vi "ICR_Hardware_Settings.vi"(8 "error in (no error)":errorcluster, 10 "Use Software Trigger":bool=TRUE, 11 "QMH UI Cluster":variant) -> (0 "error out":errorcluster, 2 "FIFO used":i64, 3 "instrument handle out":refnum<k15>)   [LabVIEW 2015]
doc: "This VI inits a waveform generation session for HSDIO 6541. This is a basic example that shows how to setup the board in order to generate waveforms according to a script. \n\n1. Initialize for a generation session.\n2. Assign specified channels in Channel List for dynamic operation : all = \"\" (default)\n3. Sets the Idle State for when the generation has completed : NO !!\n4. Configure the Sample clock to use the onboard clock, and configure the clock rate.\n5. Set generation mode to Scripted.\n6. Configure the Script Trigger : change to Digital Edge if waiting for an external\n trigger, and link Rising Edge and source trigger commands.\n Use PFI0 with SMB wired to the board, or any PFIxx if connected to accessory."
uses:
  controls/EXPERT_Inputs.ctl
  controls/SOFTWARE_Inputs.ctl
  controls/AO_6711_Inputs.ctl
  controls/AWG_5421_Inputs.ctl
  controls/DIGIT_5122_Inputs.ctl
  <instrlib>/niScope/Controls/niScope trigger source.ctl
  controls/HSDIO_6541_Inputs.ctl
  <instrlib>/niHSDIO/niHSDIO.llb/niHSDIO_ctl Trigger Source Values (Ring).ctl
  controls/SEQUENCE_Inputs.ctl
  controls/TRAPPING_Inputs.ctl
  controls/EXCIT_Inputs.ctl
  controls/DATA_Inputs.ctl
  controls/TIMING_Inputs.ctl
  controls/QMH_UI_Cluster.ctl
  controls/QMH_UI_References.ctl
  controls/QMH_UI_Report.ctl
  controls/QMH_UI_Command.ctl
  controls/QMH_ICR_Command.ctl
  controls/QMH_Status.ctl
  <instrlib>/niHSDIO/niHSDIO.llb/niHSDIO Write Named Waveform (1D U32).vi
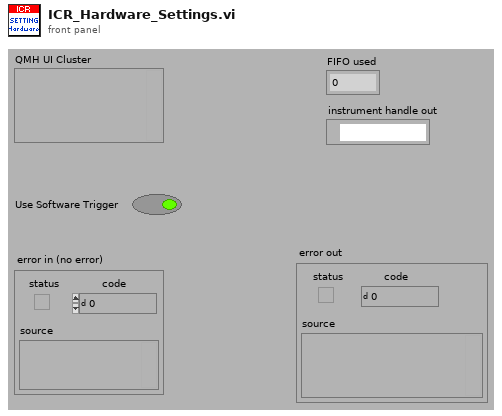
[diagram p1: front panel]
types:
  T1 = typedef "QMH_UI_Cluster.ctl" = cluster{"QMH UI References":T2, "QMH UI Report":T3}
  T2 = typedef "QMH_UI_References.ctl" = cluster{"Refnum Load":refnum<vi>, "Refnum Save":refnum<vi>, "Refnum Start":refnum<vi>, "Refnum Stop":refnum<vi>, "Refnum Exit":refnum<vi>, "Refnum Tabs":refnum<vi>, "Refnum SPECTRUM":refnum<vi>, "Refnum EXPERIMENT":refnum<vi>, "Refnum VOLTAGES":refnum<vi>, "Refnum SEQUENCE":refnum<vi>, "Refnum EXPERT":refnum<vi>, "Refnum CHANGE Experiment":refnum<vi>, "Refnum CHANGE Voltages":refnum<vi>, "Refnum CHANGE Sequence":refnum<vi>, "Refnum CHANGE Expert":refnum<vi>}
  T3 = typedef "QMH_UI_Report.ctl" = cluster{"UI Status":T4, "QLA Status":string, "ICR Status":T5, "QMH Status":T6}
  T4 = typedef "QMH_UI_Command.ctl" = enum16{"Initialize", "UI Load", "UI Save", "UI Change Experiment", "UI Change Voltages", "UI Change Sequence", "UI Change Expert", "Ready to Start", "UI Start", "UI Stop", "UI Exit", "Update Report", "Update ICR Report"}
  T5 = typedef "QMH_ICR_Command.ctl" = enum16{"Initialize", "Hardware Setup", "Waiting for Trigger", "Sequence Started", "Sequence Finished", "Writing Data", "Hardware Reset", "Exit"}
  T6 = typedef "QMH_Status.ctl" = enum16{"Init", "Loading", "Setup", "Ready to Start", "Started", "Idle"}
  T7 = typedef "SEQUENCE_Inputs.ctl" = cluster{"TRAPPING Inputs":T8, "EXCIT Inputs":T9, "DATA Inputs":T10, "TIMING Inputs":T11}
  T8 = typedef "TRAPPING_Inputs.ctl" = cluster{"Init Values":dbl[], "Opening Values":dbl[], "Trapping Values":dbl[], "Emptying Values":dbl[], "Adiabatic ON":bool, "Adiabatic Duration":i32, "Adiabatic Waveforms":string[]}
  T9 = typedef "EXCIT_Inputs.ctl" = cluster{"Number of Excitations":i32, "Table of Waveforms":string[], "Script text":string}
  T10 = typedef "DATA_Inputs.ctl" = cluster{"Record Length":i32, "Sample Rate":enum16{"1", "2", "5", "10", "20", "25", "50", "100"}, "Number of Acquisitions":i32, "Type Of Data":enum16{"I16", "DBL"}, "Vertical Range":enum16{"0.2", "0.4", "1", "2", "4", "10"}}
  T11 = typedef "TIMING_Inputs.ctl" = cluster{"Number Of Acquisitions ":i16, "Number Of Accumulations":i16, "Number Of Loops":i16, "Table of Waveforms":string[], "Script text":string}
  T12 = typedef "EXPERT_Inputs.ctl" = cluster{"SOFTWARE Inputs":T13, "AO 6711 Inputs":T14, "AWG 5421 Inputs":T15, "DIGIT 5122 Inputs":T16, "HSDIO 6541 Inputs":T18}
  T13 = typedef "SOFTWARE_Inputs.ctl" = cluster{"Application Directory":path, "Resources Path":path, "Data Path":path, "XML Path":path, "XML File Filter":string, "Excit Scripts Path":path, "Excit Scripts File Filter":string, "Excit Waveforms Path":path, "Excit Waveforms File Filter":string, "Timing Scripts Path":path, "Timing Scripts File Filter":string, "Timing Waveforms Path":path, "Timing Waveforms File Filter":string, "Trapping Waveforms Path":path, "Trapping Waveforms File Filter":string}
  T14 = typedef "AO_6711_Inputs.ctl" = cluster{"Physical Channels":tag, "Min Voltage":dbl, "Max Voltage":dbl, "Trigger Source":tag, "counter":tag}
  T15 = typedef "AWG_5421_Inputs.ctl" = cluster{"Resource Name":refnum<k15>, "Trigger Type":u16, "Trigger Source":string, "Sample Rate":dbl}
  T16 = typedef "DIGIT_5122_Inputs.ctl" = cluster{"Sample Rate":dbl, "Resource Name":refnum<k15>, "Channel Name":string, "Trigger Source":T17, "Vertical Range":dbl, "Trigger Level":dbl}
  T17 = typedef "niScope trigger source.ctl" = string
  T18 = typedef "HSDIO_6541_Inputs.ctl" = cluster{"Resource Name":refnum<k15>, "Clock Rate":dbl, "Trigger Source":T19}
  T19 = typedef "niHSDIO_ctl Trigger Source Values (Ring).ctl" = string
  T20 = enum16{"big-endian, network order", "native, host order", "little-endian"}
  T21 = enum16{"open", "replace", "create", "open or create", "replace or create", "replace or create with confirmation"}
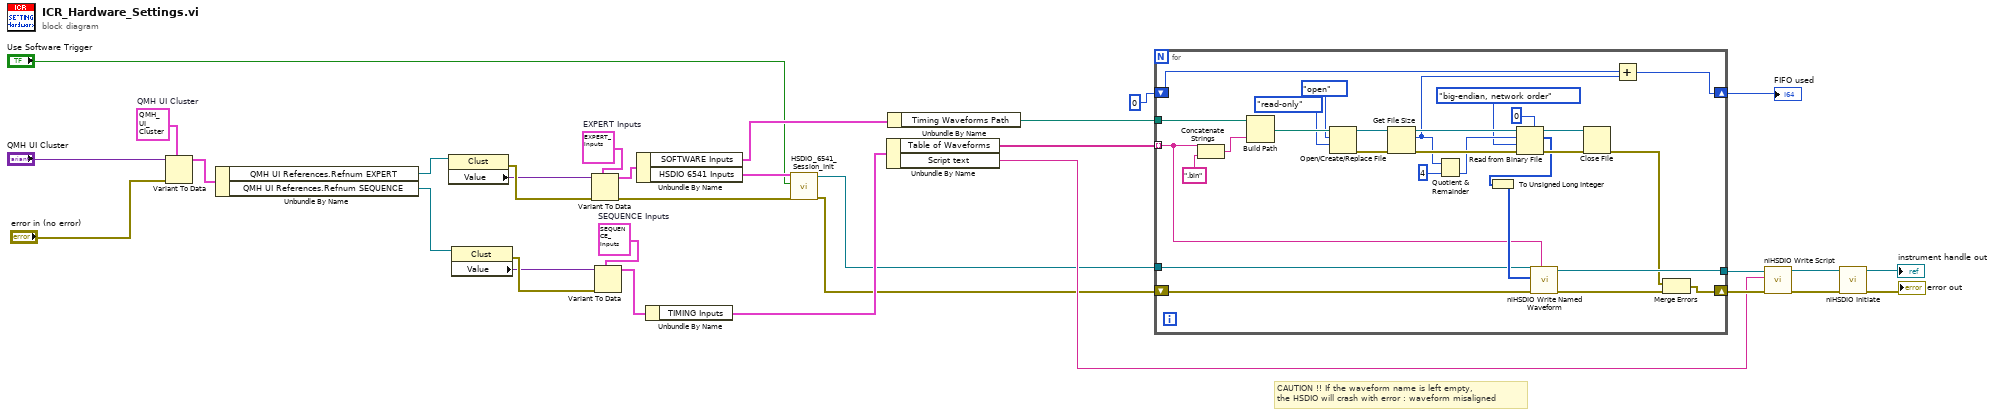
[diagram p0: block diagram]
diagram:
  w14 = T1 {"QMH UI References"={"Refnum Load"=refnum, "Refnum Save"=refnum, "Refnum Start"=refnum, "Refnum Stop"=refnum, "Refnum Exit"=refnum, "Refnum Tabs"=refnum, "Refnum SPECTRUM"=refnum, "Refnum EXPERIMENT"=refnum, "Refnum VOLTAGES"=refnum, "Refnum SEQUENCE"=refnum, "Refnum EXPERT"=refnum, "Refnum CHANGE Experiment"=refnum, "Refnum CHANGE Voltages"=refnum, "Refnum CHANGE Sequence"=refnum, "Refnum CHANGE Expert"=refnum}, "QMH UI Report"={"UI Status"=enum."Initialize", "QLA Status"="", "ICR Status"=enum."Initialize", "QMH Status"=enum."Init"}}  # QMH UI Cluster
  w27 = T7 {"TRAPPING Inputs"={"Init Values"=[2.0, 5.0, 5.0, 2.0], "Opening Values"=[0.0, 0.0, 0.0, 0.0], "Trapping Values"=[2.0, 5.0, 5.0, 2.0], "Emptying Values"=[-5.0, -5.0, -5.0, -5.0], "Adiabatic ON"=FALSE, "Adiabatic Duration"=0, "Adiabatic Waveforms"=["Adiabatic_None_2_2_2000.bin", "Adiabatic_Ramp_5_0_2000.bin", "Adiabatic_DoubleRamp_5_0_2000.bin", "Adiabatic_RC_2_0_2000.bin"]}, "EXCIT Inputs"={"Number of Excitations"=1, "Table of Waveforms"=[], "Script text"=""}, "DATA Inputs"={"Record Length"=8192, "Sample Rate"=enum."5", "Number of Acquisitions"=1, "Type Of Data"=enum."DBL", "Vertical Range"=enum."0.2"}, "TIMING Inputs"={"Number Of Acquisitions "=32767, "Number Of Accumulations"=1, "Number Of Loops"=0, "Table of Waveforms"=[], "Script text"=""}}  # SEQUENCE Inputs
  w32 = T12 {"SOFTWARE Inputs"={"Application Directory"=path "D:/S.O.F.T.S/LABVIEW/PIL", "Resources Path"=path "D:/S.O.F.T.S/LABVIEW/PIL/resources", "Data Path"=path "D:/PIRENEA/DATA", "XML Path"=path "D:/PIRENEA/DATA", "XML File Filter"="*.xml", "Excit Scripts Path"=path "D:/PIRENEA/EXCIT_SCRIPTS", "Excit Scripts File Filter"="*.txt", "Excit Waveforms Path"=path "D:/PIRENEA/EXCIT_WFMS", "Excit Waveforms File Filter"="*.bin", "Timing Scripts Path"=path "D:/PIRENEA/SEQUENCE_SCRIPTS", "Timing Scripts File Filter"="*.txt", "Timing Waveforms Path"=path "D:/PIRENEA/SEQUENCE_WFMS", "Timing Waveforms File Filter"="*.bin", "Trapping Waveforms Path"=path "D:/PIRENEA/TRAPPING_WFMS", "Trapping Waveforms File Filter"="*.bin"}, "AO 6711 Inputs"={"Physical Channels"="AnalogOutput/ao0:3", "Min Voltage"=-10.0, "Max Voltage"=10.0, "Trigger Source"="/AnalogOutput/PFI0", "counter"="AnalogOutput/ctr0"}, "AWG 5421 Inputs"={"Resource Name"="WaveformGenerator", "Trigger Type"=2, "Trigger Source"="PFI0", "Sample Rate"=20000000.0}, "DIGIT 5122 Inputs"={"Sample Rate"=10000000.0, "Resource Name"="Digitizer", "Channel Name"="0", "Trigger Source"="VAL_EXTERNAL", "Vertical Range"=10.0, "Trigger Level"=3.0}, "HSDIO 6541 Inputs"={"Resource Name"="SequencerHSDIO", "Clock Rate"=1000000.0, "Trigger Source"="PFI0"}}  # EXPERT Inputs
  # "CAUTION !! If the waveform name is left empty,\nthe HSDIO will crash with error : waveform misaligned"
  n1 = Variant To Data(error in="error in (no error)", type=w14, Variant="QMH UI Cluster") -> (data=w13:T1)  [unwired: 1 out]
  n2 = Unbundle By Name(w13) -> ("QMH UI References.Refnum EXPERT"=w12:refnum<vi>, "QMH UI References.Refnum SEQUENCE"=w11:refnum<vi>)
  n3 = property class="Clust"(reference=w12) -> (error out=w30:errorcluster, "Value"=w10:variant)  [unwired: 1 in, 1 out]
  n4 = property class="Clust"(reference=w11) -> (error out=w29:errorcluster, "Value"=w9:variant)  [unwired: 1 in, 1 out]
  n5 = Variant To Data(error in=w30, type=w32, Variant=w10) -> (data=w31:T12, error out=w6:errorcluster)
  n6 = Variant To Data(error in=w29, type=w27, Variant=w9) -> (data=w28:T7)  [unwired: 1 out]
  n7 = Unbundle By Name(w31) -> ("SOFTWARE Inputs"=w26:T13, "HSDIO 6541 Inputs"=w8:T18)
  n8 = Unbundle By Name(w28) -> ("TIMING Inputs"=w25:T11)
  n9 = call "HSDIO_6541_Session_Init.vi"("error in (no error)"=w6, "Use Software Trigger"="Use Software Trigger", "HSDIO 6541 Inputs"=w8) -> ("error out"=w5:errorcluster, "instrument handle out"=w4:refnum<k15>)  [unwired: 7 in]
  n10 = Unbundle By Name(w25) -> ("Table of Waveforms"=w21:string[], "Script text"=w20:string)
  n11 = Unbundle By Name(w26) -> ("Timing Waveforms Path"=w22:path)
  n12 = for {
    shift-right: [w38] -> w23
    shift-left: w5 -> [w45]
    shift-right: [w42] -> w17
    shift-left: i64 0 -> [w41]
    tunnel: w22 -> [w35]
    tunnel: w21 -> [w34] mode=indexing
    tunnel: [w44] -> w24
    tunnel: w4 -> [w33]
    n13 = Concatenate Strings(w34, ".bin" ("chaîne")) -> (w36:string)
    n14 = Build Path(base path=w35, name or relative path=w36) -> (appended path=w58:path)
    n15 = Open/Create/Replace File(file path (use dialog)=w58, operation (0:open)=T21."open", access (0:read/write)=enum16{"read/write", "read-only", "write-only"}."read-only") -> (refnum out=w60:refnum<file>, error out=w59:errorcluster)  [unwired: 3 in, 1 out]
    n16 = Get File Size(file=w60, error in=w59) -> (refnum out=w54:refnum<file>, size (in bytes)=w43:i64, 0:w52:errorcluster)
    n17 = Quotient & Remainder(x=w43, y=i64 4 ("type size (bytes)")) -> (floor(x/y)=w50:i64)  [unwired: 1 out]
    n18 = Read from Binary File(5:0 ("data type"), 8:w52, 9:T20."big-endian, network order" ("ordre des octets (0 : big-Endian, network order)"), 10:w50, 11:w54) -> (0:w51:errorcluster, 2:w47:i32[], 3:w53:refnum<file>)  [unwired: 1 in, 1 out]
    n19 = To Unsigned Long Integer(number=w47) -> (unsigned 32bit integer=w49:u32[])
    n20 = call-poly <instrlib>:"niHSDIO Write Named Waveform.vi"("waveform name (default:\"\")"=w34, "error in (no error)"=w45, "data"=w49, "instrument handle"=w33) -> ("error out"=w39:errorcluster, "instrument handle out"=w44:refnum<k15>)  [unwired: 6 in]
    n21 = Close File(refnum=w53, error in=w51) -> (error out=w40:errorcluster)  [unwired: 1 out]
    n22 = Add(x=w41, y=w43) -> (x+y=w42:i64)
    n23 = Merge Errors(w40, w39) -> (w38:errorcluster)
  }
  "FIFO used" <- w17
  n24 = call <instrlib>:"niHSDIO Write Script.vi"("error in (no error)"=w23, "script"=w20, "instrument handle"=w24) -> ("error out"=w18:errorcluster, "instrument handle out"=w19:refnum<k15>)  [unwired: 7 in]
  n25 = call <instrlib>:"niHSDIO Initiate.vi"("error in (no error)"=w18, "instrument handle"=w19) -> ("error out"=→"error out":errorcluster, "instrument handle out"=→"instrument handle out":refnum<k15>)  [unwired: 8 in]
